vi "process_analysis.vi"(8 "error in (no error)":errorcluster) -> (0 "error out":errorcluster)   [LabVIEW 2010]
uses:
  typedefs/analysis_cluster_dual_channel.ctl
  typedefs/analysis_cluster.ctl
  typedefs/control_analysis_enum.ctl
  typedefs/data_cluster.ctl
  typedefs/experiment_mode_enum.ctl
panel:
  in  "What to store":enum32{"Raw data", "Analyzed data"}(radio)
  out "Analysis":T1
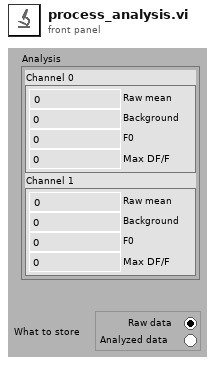
[diagram p1: front panel]
types:
  T1 = typedef "analysis_cluster_dual_channel.ctl" = cluster{"Channel 0":T2, "Channel 1":T2}
  T2 = typedef "analysis_cluster.ctl" = cluster{"Raw mean":dbl, "Background":dbl, "F0":dbl, "Max DF/F":dbl}
  T3 = typedef "data_cluster.ctl" = cluster{"t0":dbl, "dt":dbl, "Channels":dbl[][]}
  T4 = typedef "control_analysis_enum.ctl" = enum16{"Init", "Analyze", "Reset", "Stop", "Quit"}
  T5 = cluster{"Control Analysis Enum":T4, "variant":variant}
  T6 = cluster{"Data_to_Display_Queue":refnum<queue>, "Data_to_Storage_Queue":refnum<queue>}
  T7 = typedef "experiment_mode_enum.ctl" = enum32{"Raw data", "Measure background", "Measure F0", "Measure DF/F"}
  T8 = cluster{"Experiment mode":T7, "Pixels to integrate":i32, "#channels":i32, "Iteration":i32}
  T9 = typedef "analysis_channels_array.ctl" = T2[]
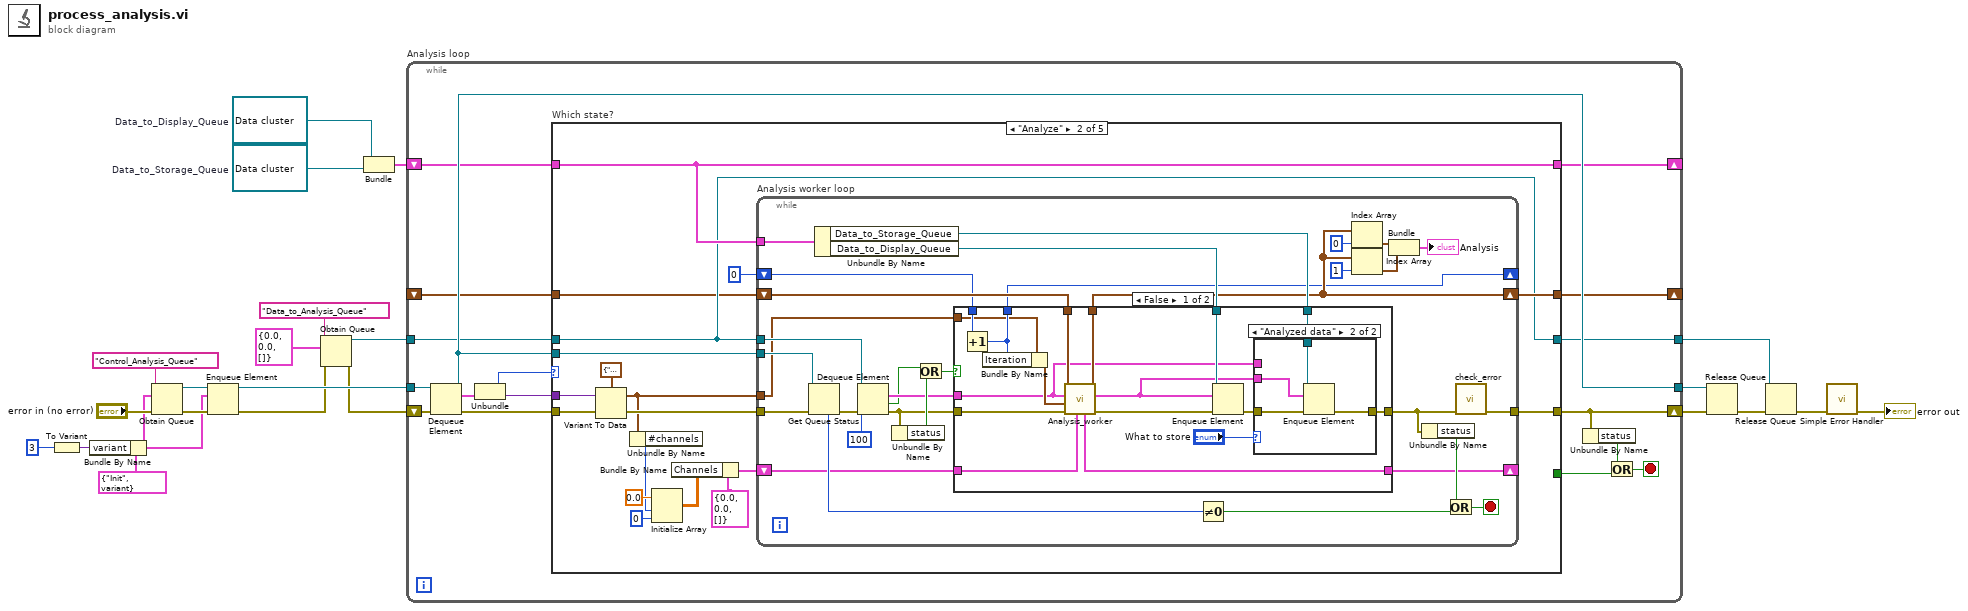
[diagram p0: block diagram]
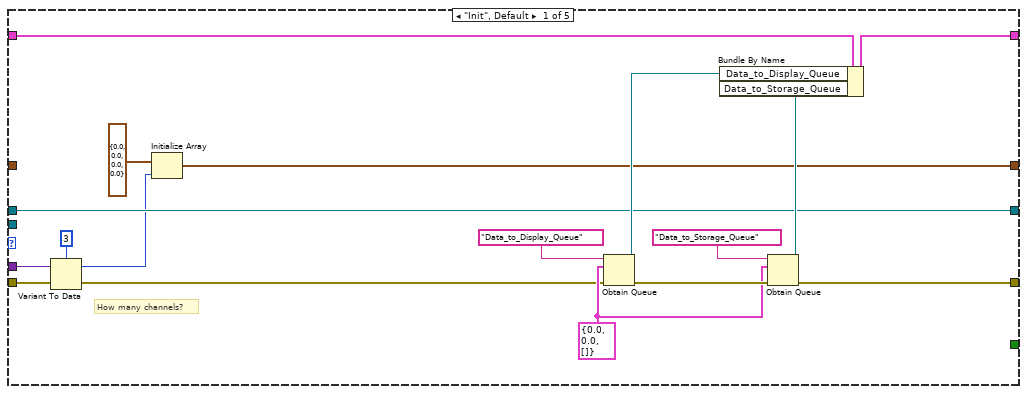
[diagram p2: hidden frame]
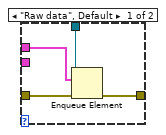
[diagram p3: hidden frame]
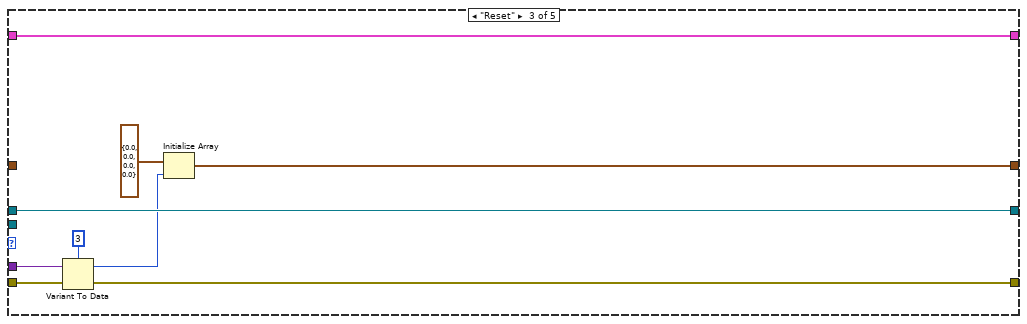
[diagram p5: hidden frame]
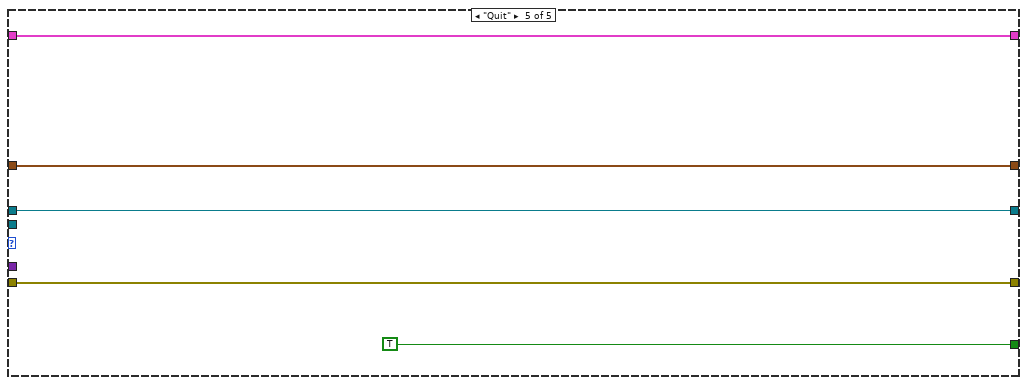
[diagram p7: hidden frame]
diagram:
  w7 = refnum<queue> refnum  # Data_to_Storage_Queue
  w8 = refnum<queue> refnum  # Data_to_Display_Queue
  n1 = To Variant(anything=3) -> (Variant=w2:variant)
  n2 = Bundle By Name(cluster=T5 {"Control Analysis Enum"=enum."Init", "variant"=variant}, "variant"=w2) -> (w1:T5)
  n3 = Obtain Queue(name (unnamed)="Control_Analysis_Queue", element data type=w1, error in (no error)="error in (no error)") -> (queue out=w20:refnum<queue>, error out=w21:errorcluster)  [unwired: 2 in, 1 out]
  n4 = Enqueue Element(queue=w20, element=w1, error in (no error)=w21) -> (queue out=w19:refnum<queue>, error out=w15:errorcluster)  [unwired: 1 in, 1 out]
  n5 = Obtain Queue(name (unnamed)="Data_to_Analysis_Queue", element data type=T3 {"t0"=0.0, "dt"=0.0, "Channels"=[]} ("Data cluster"), error in (no error)=w15) -> (queue out=w13:refnum<queue>, error out=w14:errorcluster)  [unwired: 2 in, 1 out]
  n6 = Bundle("Data_to_Display_Queue"=w8, "Data_to_Storage_Queue"=w7) -> (w12:T6)  [unwired: 1 in]
  n7 = while "Analysis loop" {
    shift-right: [w35] -> w18
    shift-left: w14 -> [w37]
    tunnel: w19 -> [w38]
    tunnel: [w30] -> w17
    tunnel: w13 -> [w24]
    shift-right: [w28] -> _
    shift-left: w12 -> [w29]
    tunnel: [w27] -> w10
    shift-right: [w25] -> _
    shift-left: _ -> [w26]
    stop <- w39 stop-if-true
    n8 = Dequeue Element(queue=w38, error in (no error)=w37) -> (queue out=w30:refnum<queue>, element=w34:T5, error out=w36:errorcluster)  [unwired: 1 in, 1 out]
    n9 = Unbundle(w34) -> ("Control Analysis Enum"=w33:T4, "variant"=w32:variant)
    n10 = case "Which state?" shown="\"Analyze\"" w33 {
      tunnel: w36 -> [w46 w72 w140 w148 w153]
      tunnel: [w53 w75 w139 w148 w153] -> w35
      tunnel: w32 -> [w44 w70 w138 _ _]
      tunnel: [_ _ _ _ TRUE] -> w31
      tunnel: w30 -> [_ w74 _ _ _]
      tunnel: w29 -> [w56 w73 w144 w147 w151]
      tunnel: [w55 w73 w144 w147 w151] -> w28
      tunnel: [w49 w66 w143 w146 w150] -> w27
      tunnel: w26 -> [_ w58 _ w145 w149]
      tunnel: [w41 w69 w136 w145 w149] -> w25
      tunnel: w24 -> [w49 w66 w143 w146 w150]
      frame "Init", Default {
        w48 = T3 {"t0"=0.0, "dt"=0.0, "Channels"=[]} ("Data cluster")
        # "How many channels?"
        n11 = Variant To Data(error in=w46, Variant=w44, type=3) -> (error out=w45:errorcluster, data=w42:i32)
        n12 = Initialize Array(T2 {"Raw mean"=0.0, "Background"=0.0, "F0"=0.0, "Max DF/F"=0.0} ("Analysis"), w42) -> (w41:T2[])
        n13 = Obtain Queue(name (unnamed)="Data_to_Display_Queue", element data type=w48, error in (no error)=w45) -> (queue out=w51:refnum<queue>, error out=w54:errorcluster)  [unwired: 2 in, 1 out]
        n14 = Obtain Queue(name (unnamed)="Data_to_Storage_Queue", element data type=w48, error in (no error)=w54) -> (queue out=w50:refnum<queue>, error out=w53:errorcluster)  [unwired: 2 in, 1 out]
        n15 = Bundle By Name(cluster=w56, "Data_to_Display_Queue"=w51, "Data_to_Storage_Queue"=w50) -> (w55:T6)
      }
      frame "Analyze" {
        n16 = Variant To Data(error in=w72, Variant=w70, type=T8 {"Experiment mode"=enum."Raw data", "Pixels to integrate"=0, "#channels"=0, "Iteration"=0} ("output cluster")) -> (error out=w71:errorcluster, data=w63:T8)
        n17 = Unbundle By Name(w63) -> ("#channels"=w59:i32)
        n18 = Initialize Array(0.0 ("element"), w59, 0 ("dimension size")) -> (w60:dbl[][])
        n19 = Bundle By Name(cluster=T3 {"t0"=0.0, "dt"=0.0, "Channels"=[]} ("Leftover data out"), "Channels"=w60) -> (w64:T3)
        n20 = while "Analysis worker loop" {
          tunnel: w71 -> [w105]
          tunnel: [w78] -> w75
          tunnel: w74 -> [w103]
          tunnel: w73 -> [w98]
          tunnel: w66 -> [w106]
          tunnel: w63 -> [w82]
          shift-right: [w92] -> w69
          shift-left: w58 -> [w95]
          shift-right: [w93] -> _
          shift-left: w64 -> [w94]
          shift-right: [w80] -> _
          shift-left: 0 -> [w81]
          stop <- w99 stop-if-true
          n21 = Get Queue Status(queue=w103, error in (no error)=w105) -> (error out=w104:errorcluster, # elements in queue=w102:i32)  [unwired: 1 in, 6 out]
          n22 = Unbundle By Name(w98) -> ("Data_to_Storage_Queue"=w96:refnum<queue>, "Data_to_Display_Queue"=w97:refnum<queue>)
          n23 = Dequeue Element(queue=w106, timeout in ms (-1)=100, error in (no error)=w104) -> (element=w77:T3, timed out?=w76:bool, error out=w83:errorcluster)  [unwired: 1 out]
          n24 = Unbundle By Name(w83) -> ("status"=w85:bool)
          n25 = Or(x=w76, y=w85) -> (x .or. y?=w84:bool)
          n26 = case shown="False" w84 {
            tunnel: [w123 w133] -> w79
            tunnel: w97 -> [w122 _]
            tunnel: w96 -> [w121 _]
            tunnel: [w120 w135] -> w92
            tunnel: w95 -> [w119 w135]
            tunnel: w94 -> [w115 w134]
            tunnel: [w114 w134] -> w93
            tunnel: w82 -> [w110 _]
            tunnel: w83 -> [w113 w133]
            tunnel: w81 -> [w112 w132]
            tunnel: [w111 w132] -> w80
            tunnel: w77 -> [w108 _]
            frame False {
              n27 = Increment(x=w112) -> (x+1=w111:i32)
              n28 = Bundle By Name(cluster=w110, "Iteration"=w111) -> (w109:T8)
              n29 = call "Analysis_worker.vi"("Leftover data in"=w115, "error in"=w113, "Analysis parameters"=w109, "Data in"=w108, "Analysis in"=w119) -> ("error out"=w117:errorcluster, "Data out"=w107:T3, "Analysis out"=w120:T9, "Leftover data out"=w114:T3)  [unwired: 1 in]
              n30 = Enqueue Element(queue=w122, element=w107, error in (no error)=w117) -> (error out=w118:errorcluster)  [unwired: 1 in, 2 out]
              n31 = case shown="\"Analyzed data\"" "What to store" {
                tunnel: [w126 w131] -> w123
                tunnel: w121 -> [w125 w130]
                tunnel: w118 -> [w127 w129]
                tunnel: w108 -> [w124 _]
                tunnel: w107 -> [_ w128]
                frame "Raw data", Default {
                  n32 = Enqueue Element(queue=w125, element=w124, error in (no error)=w127) -> (error out=w126:errorcluster)  [unwired: 1 in, 2 out]
                }
                frame "Analyzed data" {
                  n33 = Enqueue Element(queue=w130, element=w128, error in (no error)=w129) -> (error out=w131:errorcluster)  [unwired: 1 in, 2 out]
                }
              }
            }
            frame True {
            }
          }
          n34 = Not Equal To 0?(x=w102) -> (x != 0?=w101:bool)
          n35 = Index Array(array=w92, index=0) -> (element=w88:T2)
          n36 = Index Array(array=w92, index=1) -> (element=w87:T2)
          n37 = Bundle("Analysis"=w88, "Analysis"=w87) -> (→"Analysis":cluster{"Analysis":T2, "Analysis":T2})  [unwired: 1 in]
          n38 = Unbundle By Name(w79) -> ("status"=w100:bool)
          n39 = Or(x=w100, y=w101) -> (x .or. y?=w99:bool)
          n40 = call "check_error.vi"("error in"=w79) -> ("error out"=w78:errorcluster)  [unwired: 10 in]
        }
      }
      frame "Reset" {
        n41 = Variant To Data(error in=w140, Variant=w138, type=3) -> (error out=w139:errorcluster, data=w141:i32)
        n42 = Initialize Array(T2 {"Raw mean"=0.0, "Background"=0.0, "F0"=0.0, "Max DF/F"=0.0} ("Analysis"), w141) -> (w136:T2[])
      }
      frame "Stop" {
      }
      frame "Quit" {
      }
    }
    n43 = Unbundle By Name(w35) -> ("status"=w40:bool)
    n44 = Or(x=w40, y=w31) -> (x .or. y?=w39:bool)
  }
  n45 = Release Queue(queue=w17, error in (no error)=w18) -> (error out=w11:errorcluster)  [unwired: 1 in, 2 out]
  n46 = Release Queue(queue=w10, error in (no error)=w11) -> (error out=w6:errorcluster)  [unwired: 1 in, 2 out]
  n47 = call <vilib>:"Simple Error Handler.vi"("error in (no error)"=w6) -> ("error out"=→"error out":errorcluster)  [unwired: 4 in, 4 out]
